vi "Open_Close_Front_Panel.ph.vi"(1 "runVI (F)":bool, 2 "openWindow (T)":bool=TRUE, 3 "VI path":path) -> (0 "error out":errorcluster)   [LabVIEW 2021]
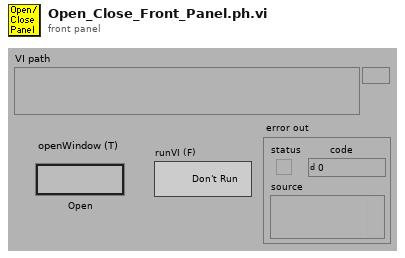
[diagram p1: front panel]
types:
  T1 = enum32{"Invalid", "Standard", "Closed", "Hidden", "Minimized", "Maximized"}
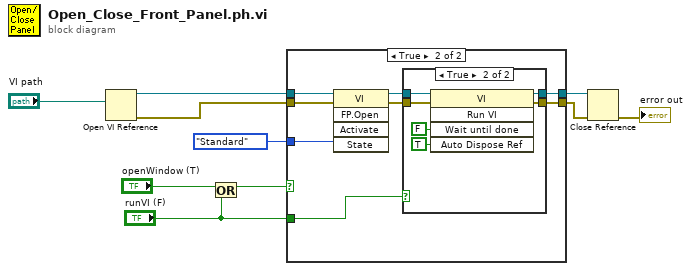
[diagram p0: block diagram]
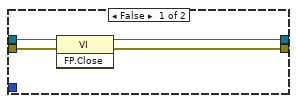
[diagram p2: hidden frame]
diagram:
  n1 = Open VI Reference(vi path="VI path") -> (vi reference=w6:refnum<vi>, error out=w8:errorcluster)  [unwired: 1 in, 4 out]
  n2 = Or(x="openWindow (T)", y="runVI (F)") -> (x .or. y?=w2:bool)
  n3 = case shown="True" w2 {
    tunnel: w8 -> [w11 w21]
    tunnel: [w12 w16] -> w7
    tunnel: w6 -> [w14 w22]
    tunnel: [w13 w17] -> w5
    tunnel: T1."Standard" ("State") -> [_ w20]
    tunnel: "runVI (F)" -> [_ w15]
    frame False {
      n4 = invoke class="VI" method="FP.Close"(reference=w14, error in=w11) -> (reference out=w13:refnum<vi>, error out=w12:errorcluster)  [unwired: 1 in, 1 out]
    }
    frame True {
      n5 = invoke class="VI" method="FP.Open"(reference=w22, error in=w21, "State"=w20) -> (reference out=w19:refnum<vi>, error out=w18:errorcluster)  [unwired: 2 in, 3 out]
      n6 = case shown="True" w15 {
        tunnel: w19 -> [w24 w28]
        tunnel: w18 -> [w23 w27]
        tunnel: [w24 w26] -> w17
        tunnel: [w23 w25] -> w16
        frame False {
        }
        frame True {
          n7 = invoke class="VI" method="Run VI"(reference=w28, error in=w27, "Wait until done"=FALSE ("Wait Until Done"), "Auto Dispose Ref"=TRUE ("Wait Until Done")) -> (reference out=w26:refnum<vi>, error out=w25:errorcluster)  [unwired: 1 in, 3 out]
        }
      }
    }
  }
  n8 = Close Reference(reference=w5, error in (no error)=w7) -> (error out=→"error out":errorcluster)
